vi "Initialize and Functional.vi"() -> ()   [LabVIEW 2024]
uses:
  <vilib>/Instr/_visa.llb/VISA Configure Serial Port (Instr).vi
panel:
  out "connection information":path
  in  "Exit":bool
  in  "Initialize Boards":bool
  out "TITLE":string
  out "System Number":string
  out "Time":string
  out "System Status":string
  out "Functional Test Data":string
  in  "Functional Test":bool
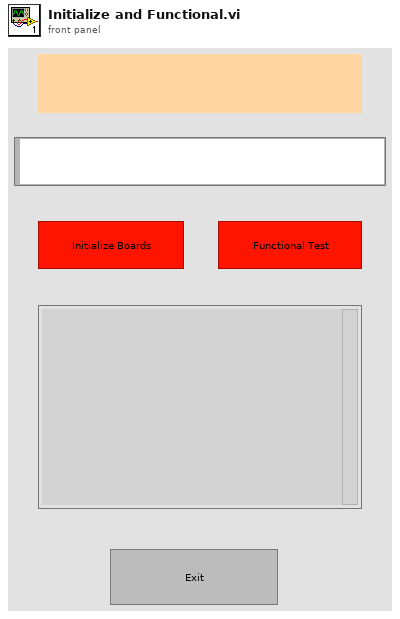
[diagram p1: front panel]
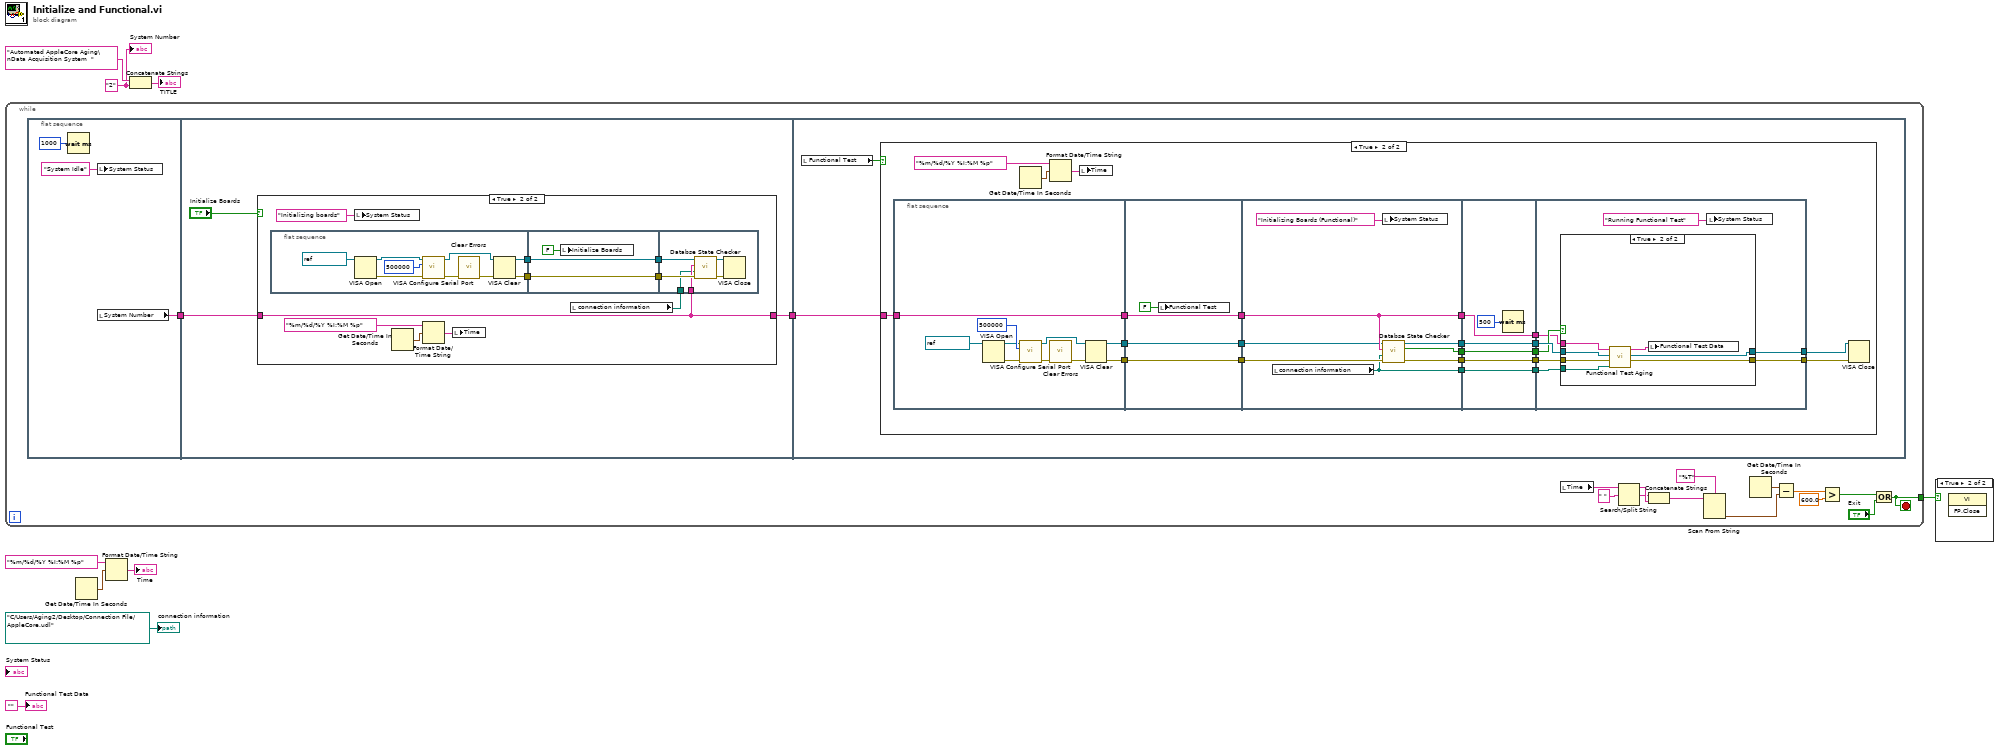
[diagram p0: block diagram]
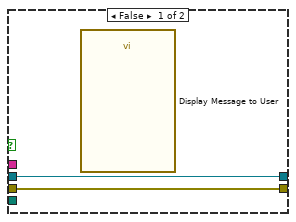
[diagram p5: hidden frame]
diagram:
  w3 = "2" ("substring")
  n1 = while {
    tunnel: [w10] -> w2
    stop <- w10 stop-if-true
    n2 = flat-sequence {
      tunnel: [w25] -> w14
      tunnel: w14 -> [w30]
      tunnel: [w28] -> w13
      tunnel: w13 -> [w60]
      frame #0 {
        n3 = Wait (ms)(milliseconds to wait=u32 1000) -> ()  [unwired: 1 out]
        n4 = local write "System Status"("System Idle" ("System Status")) -> ()
        n5 = local read "System Number"() -> (w25:string)
      }
      frame #1 {
        n6 = case shown="True" "Initialize Boards" {
          tunnel: w30 -> [w31 w33]
          tunnel: [w31 w33] -> w28
          frame False {
          }
          frame True {
            n7 = flat-sequence {
              tunnel: [w43] -> w37
              tunnel: [w42] -> w36
              tunnel: w37 -> [w53]
              tunnel: w36 -> [w52]
              tunnel: [w53] -> w35
              tunnel: [w52] -> w34
              tunnel: w35 -> [w55]
              tunnel: w34 -> [w57]
              tunnel: w33 -> [w56]
              tunnel: w32 -> [w54]
              frame #0 {
                n8 = VISA Open(VISA resource name=refnum<visa-resource-name> "COM4") -> (VISA resource name=w47:refnum<visa-resource-name>, error out=w48:errorcluster)  [unwired: 4 in]
                n9 = call-poly "VISA Configure Serial Port"("VISA resource name"=w47, "baud rate (9600)"=u32 500000, "error in (no error)"=w48) -> ("VISA resource name out"=w49:refnum<visa-resource-name>, "error out"=w50:errorcluster)  [unwired: 11 in]
                n10 = call <vilib>:"Clear Errors.vi"("error in (no error)"=w50) -> ("error out"=w46:errorcluster)  [unwired: 5 in, 1 out]
                n11 = VISA Clear(VISA resource name=w49, error in (no error)=w46) -> (VISA resource name out=w43:refnum<visa-resource-name>, error out=w42:errorcluster)
              }
              frame #1 {
                n12 = local write "Initialize Boards"(FALSE ("Initialize Boards")) -> ()
              }
              frame #2 {
                n13 = call "Databse State Checker.vi"("error in (no error)"=w57, "connection information"=w54, "System Number"=w56, "Arduino in"=w55) -> ("error out"=w59:errorcluster, "Arduino out"=w58:refnum<visa-resource-name>)  [unwired: 5 in, 1 out]
                n14 = VISA Close(VISA resource name=w58, error in (no error)=w59) -> ()  [unwired: 1 out]
              }
            }
            n15 = local write "System Status"("Initializing boards" ("System Status")) -> ()
            n16 = Get Date/Time In Seconds() -> (seconds since 1Jan1904=w40:timestamp)
            n17 = Format Date/Time String(time format string (%c)="%m/%d/%Y %I:%M %p", seconds (now)=w40) -> (date/time string=w39:string)  [unwired: 1 in]
            n18 = local write "Time"(w39) -> ()
            n19 = local read "connection information"() -> (w32:path)
          }
        }
      }
      frame #2 {
        n20 = local read "Functional Test"() -> (w61:bool)
        n21 = case shown="True" w61 {
          tunnel: w60 -> [_ w81]
          frame False {
          }
          frame True {
            n22 = flat-sequence {
              tunnel: w81 -> [w86]
              tunnel: [w86] -> w69
              tunnel: [w85] -> w66
              tunnel: [w84] -> w64
              tunnel: w69 -> [w97]
              tunnel: [w97] -> w68
              tunnel: [w96] -> w67
              tunnel: w66 -> [w96]
              tunnel: [w95] -> w65
              tunnel: w64 -> [w95]
              tunnel: [w100] -> w73
              tunnel: [w102] -> w72
              tunnel: [w101] -> w71
              tunnel: w68 -> [w104]
              tunnel: [w104] -> w70
              tunnel: w67 -> [w105]
              tunnel: w65 -> [w103]
              tunnel: [w98] -> w62
              tunnel: [w110] -> w83
              tunnel: [w109] -> w82
              tunnel: w73 -> [w110]
              tunnel: w72 -> [w109]
              tunnel: w71 -> [w108]
              tunnel: [w108] -> w78
              tunnel: [w107] -> w77
              tunnel: w70 -> [w107]
              tunnel: [w106] -> w63
              tunnel: w62 -> [w106]
              tunnel: w83 -> [w118]
              tunnel: w82 -> [w119]
              tunnel: [w117] -> w80
              tunnel: [w116] -> w79
              tunnel: w78 -> [w115]
              tunnel: w77 -> [w114]
              tunnel: w63 -> [w112]
              frame #0 {
                n23 = VISA Open(VISA resource name=refnum<visa-resource-name> "COM4") -> (VISA resource name=w89:refnum<visa-resource-name>, error out=w92:errorcluster)  [unwired: 4 in]
                n24 = call-poly "VISA Configure Serial Port"("VISA resource name"=w89, "baud rate (9600)"=u32 500000, "error in (no error)"=w92) -> ("VISA resource name out"=w88:refnum<visa-resource-name>, "error out"=w93:errorcluster)  [unwired: 11 in]
                n25 = call <vilib>:"Clear Errors.vi"("error in (no error)"=w93) -> ("error out"=w91:errorcluster)  [unwired: 5 in, 1 out]
                n26 = VISA Clear(VISA resource name=w88, error in (no error)=w91) -> (VISA resource name out=w84:refnum<visa-resource-name>, error out=w85:errorcluster)
              }
              frame #1 {
                n27 = local write "Functional Test"(FALSE ("Functional Test")) -> ()
              }
              frame #2 {
                n28 = local read "connection information"() -> (w98:path)
                n29 = local write "System Status"("Initializing Boards (Functional)" ("System Status")) -> ()
                n30 = call "Databse State Checker.vi"("error in (no error)"=w105, "connection information"=w98, "System Number"=w104, "Arduino in"=w103) -> ("error out"=w102:errorcluster, "Database Available?"=w101:bool, "Arduino out"=w100:refnum<visa-resource-name>)  [unwired: 5 in]
              }
              frame #3 {
                n31 = Wait (ms)(milliseconds to wait=u32 500) -> ()  [unwired: 1 out]
              }
              frame #4 {
                n32 = case shown="True" w115 {
                  tunnel: w119 -> [w120 w128]
                  tunnel: w118 -> [w121 w127]
                  tunnel: w114 -> [_ w126]
                  tunnel: [w120 w125] -> w117
                  tunnel: [w121 w124] -> w116
                  tunnel: w112 -> [_ w122]
                  frame False {
                    n33 = call "Display Message to User"() -> ()  [unwired: 10 in, 2 out]
                  }
                  frame True {
                    n34 = call "Functional Test Aging.vi"("connection information"=w122, "error in"=w128, "Arduino"=w127, "System Number"=w126) -> ("error out"=w125:errorcluster, "Arduino"=w124:refnum<visa-resource-name>, "Functional Test Data"=w123:string)  [unwired: 5 in]
                    n35 = local write "Functional Test Data"(w123) -> ()
                  }
                }
                n36 = local write "System Status"("Running Functional Test" ("System Status")) -> ()
              }
            }
            n37 = Get Date/Time In Seconds() -> (seconds since 1Jan1904=w76:timestamp)
            n38 = Format Date/Time String(time format string (%c)="%m/%d/%Y %I:%M %p", seconds (now)=w76) -> (date/time string=w74:string)  [unwired: 1 in]
            n39 = local write "Time"(w74) -> ()
            n40 = VISA Close(VISA resource name=w79, error in (no error)=w80) -> ()  [unwired: 1 out]
          }
        }
      }
    }
    n41 = local read "Time"() -> (w20:string)
    n42 = Search/Split String(string=w20, search string/char (-)=" ") -> (substring before match=w22:string, match + rest of string=w21:string)  [unwired: 1 in, 1 out]
    n43 = Concatenate Strings(w21, w22) -> (w19:string)
    n44 = Scan From String(format string="%T", input string=w19) -> (output 1=w12:timestamp)  [unwired: 3 in, 3 out]
    n45 = Get Date/Time In Seconds() -> (seconds since 1Jan1904=w11:timestamp)
    n46 = Subtract(x=w11, y=w12) -> (x-y=w18:dbl)
    n47 = Greater?(x=w18, y=600.0) -> (0:w15:bool)
    n48 = Or(x=w15, y="Exit") -> (x .or. y?=w10:bool)
  }
  n49 = Get Date/Time In Seconds() -> (seconds since 1Jan1904=w7:timestamp)
  n50 = Format Date/Time String(time format string (%c)="%m/%d/%Y %I:%M %p", seconds (now)=w7) -> (date/time string=→"Time":string)  [unwired: 1 in]
  n51 = Concatenate Strings("Automated AppleCore Aging\nData Acquisition System  " ("TITLE"), w3) -> (→"TITLE":string)
  n52 = case shown="True" w2 {
    frame False {
    }
    frame True {
      n53 = invoke class="VI" method="FP.Close"() -> ()  [unwired: 3 in, 3 out]
    }
  }
  "Functional Test Data" <- ""
  "System Number" <- w3
  "connection information" <- path "C:/Users/Aging2/Desktop/Connection File/AppleCore.udl" ("connection information")
